vi "Calculate AOL Z middle pos.vi"() -> (3 "AOL Z-stack middle position":dbl)   [LabVIEW 2013]
panel:
  out "Test illustration slider":cluster{dbl, dbl, dbl}(slide)={0.0, 5.357142857142857, 7.261904761904762} scale=-10.0..10.0
  in  "Use test inputs":bool
  in  "Start":dbl=8.0 min=-10.0 max=10.0
  in  "Stop":dbl=-8.0 min=-10.0 max=10.0
  # "Test Inputs"
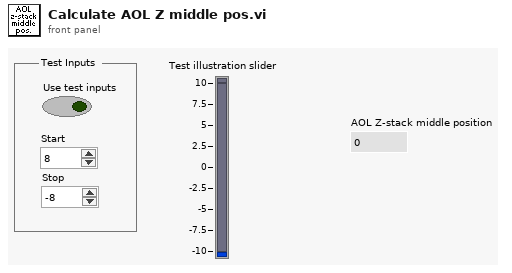
[diagram p1: front panel]
types:
  T1 = cluster{"ZStack":cluster{"Zstart":dbl, "Zstop":dbl, "Zstep":dbl}, "Laser Power %":cluster{"@ Start":dbl, "@ Stop":dbl}}
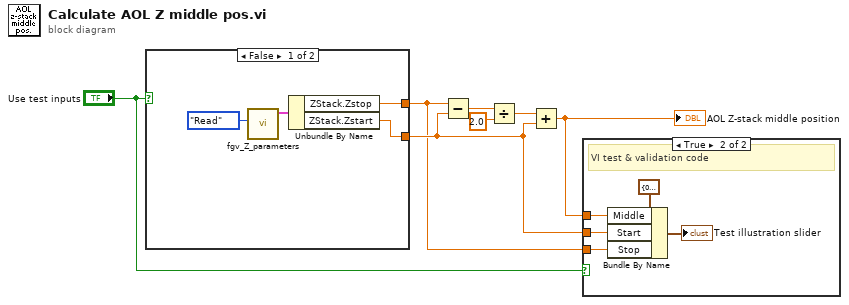
[diagram p0: block diagram]
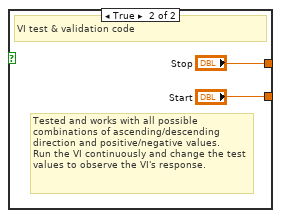
[diagram p3: hidden frame]
diagram:
  n1 = case shown="False" "Use test inputs" {
    tunnel: [w8 "Start"] -> w3
    tunnel: [w11 "Stop"] -> w2
    frame False {
      n2 = call "fgv_Z_parameters.vi"("Function"=enum16{"Intialize", "Write", "Read", "Clear"}."Read") -> ("Z Parameters"=w9:T1)  [unwired: 9 in, 1 out]
      n3 = Unbundle By Name(w9) -> ("ZStack.Zstop"=w11:dbl, "ZStack.Zstart"=w8:dbl)
    }
    frame True {
      # "Tested and works with all possible combinations of ascending/descending direction and positive/negative values.\nRun the VI continuously and change the test values to observe the VI's response."
      # "VI test & validation code"
    }
  }
  n4 = Subtract(x=w2, y=w3) -> (x-y=w6:dbl)
  n5 = Divide(x=w6, y=2.0) -> (x/y=w7:dbl)
  n6 = Add(x=w7, y=w3) -> (x+y=w4:dbl)
  "AOL Z-stack middle position" <- w4
  n7 = case shown="True" "Use test inputs" {
    tunnel: w4 -> [_ w16]
    tunnel: w3 -> [_ w15]
    tunnel: w2 -> [_ w14]
    frame False {
    }
    frame True {
      # "VI test & validation code"
      n8 = Bundle By Name(cluster=cluster{"Start":dbl, "Middle":dbl, "Stop":dbl} {"Start"=0.0, "Middle"=0.0, "Stop"=0.0} ("Test illustration slider"), "Middle"=w16, "Start"=w15, "Stop"=w14) -> (→"Test illustration slider":cluster{"Start":dbl, "Middle":dbl, "Stop":dbl})
    }
  }
